vi "Create Directory if Non-Existant.vi"(8 "error in (no error)":errorcluster, 9 "permissions (0755)":i16=493 format="%.0o", 11 "Directory Path":path) -> (0 "error out":errorcluster, 2 "Created Directories":path[](array[path]), 3 "dup Directory Path":path)   [LabVIEW 2017]
doc: "Will create all directories above and including the directory defined by the \"Directory Path\" input, if they do not already exist."
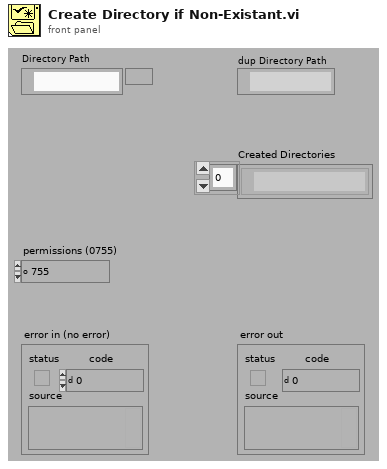
[diagram p1: front panel]
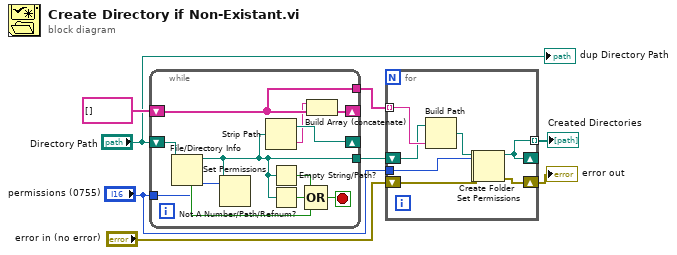
[diagram p0: block diagram]
diagram:
  n1 = while {
    shift-right: [w12] -> _
    shift-left: "Directory Path" -> [w19]
    shift-right: [w18] -> _
    shift-left: string[] [] -> [w17]
    tunnel: [w17] -> w5
    tunnel: [w10] -> w4
    tunnel: "permissions (0755)" -> [w9]
    stop <- w16 stop-if-true
    n2 = File/Directory Info(path=w19) -> (path out=w10:path, directory=w13:bool)  [unwired: 1 in, 5 out]
    n3 = Set Permissions(7:w9, 11:w10) -> ()  [unwired: 3 in, 2 out]
    n4 = Strip Path(path=w10) -> (stripped path=w12:path, name=w11:string)
    n5 = Empty String/Path?(string/path=w10) -> (empty?=w15:bool)
    n6 = Not A Number/Path/Refnum?(number/path/refnum=w10) -> (NaN/Path/Refnum?=w14:bool)
    n7 = Compound Arithmetic op=OR(w15, w14, w13) -> (w16:bool)
    n8 = Build Array (concatenate)(w11, w17) -> (w18:string[])
  }
  n9 = for {
    tunnel: w5 -> [w28] mode=indexing
    shift-right: [w22] -> _
    shift-left: w4 -> [w27]
    shift-right: [w26] -> w7
    shift-left: "error in (no error)" -> [w25]
    tunnel: "permissions (0755)" -> [w23]
    tunnel: [w22] -> w1 mode=indexing
    n10 = Build Path(base path=w27, name or relative path=w28) -> (appended path=w24:path)
    n11 = Create Folder(path (use dialog)=w24, error in=w25) -> (created path=w21:path, error out=w20:errorcluster)  [unwired: 1 in, 1 out]
    n12 = Set Permissions(7:w23, 8:w20, 11:w21) -> (0:w26:errorcluster, 3:w22:path)  [unwired: 2 in]
  }
  "error out" <- w7
  "Created Directories" <- w1
  "dup Directory Path" <- "Directory Path"
